vi "cluster2array_side_circle_overlay.vi"(10 "radius":i32, 11 "giltch of clusters":cluster{"giltch_coord":dbl[]}[](array[cluster])) -> (0 "Left side points":T1, 1 "Bottom side points":T1, 2 "Right side points":T1, 3 "Top side points":T1)   [LabVIEW 2017]
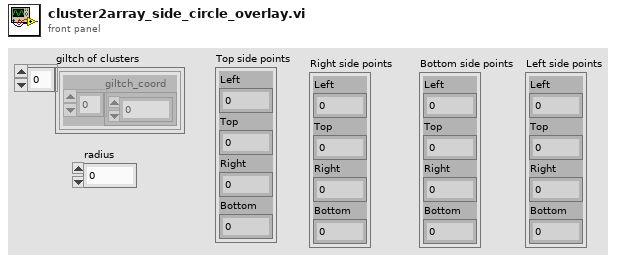
[diagram p1: front panel]
types:
  T1 = cluster{"Left":i32, "Top":i32, "Right":i32, "Bottom":i32}
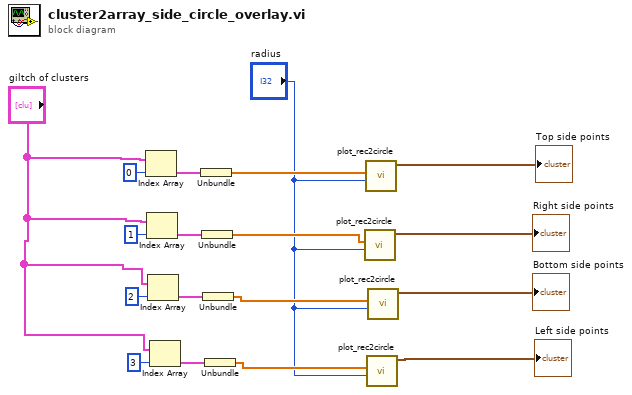
[diagram p0: block diagram]
diagram:
  n1 = Index Array(array="giltch of clusters", index=0 ("index (page)")) -> (element=w17:cluster{"giltch_coord":dbl[]})
  n2 = Index Array(array="giltch of clusters", index=1 ("index (page)")) -> (element=w14:cluster{"giltch_coord":dbl[]})
  n3 = Index Array(array="giltch of clusters", index=2 ("index (page)")) -> (element=w13:cluster{"giltch_coord":dbl[]})
  n4 = Index Array(array="giltch of clusters", index=3 ("index (page)")) -> (element=w10:cluster{"giltch_coord":dbl[]})
  n5 = Unbundle(w17) -> ("giltch_coord"=w8:dbl[])
  n6 = Unbundle(w14) -> ("giltch_coord"=w7:dbl[])
  n7 = Unbundle(w13) -> ("giltch_coord"=w6:dbl[])
  n8 = Unbundle(w10) -> ("giltch_coord"=w5:dbl[])
  n9 = call "plot_rec2circle.vi"("radius"="radius", "center of circle"=w7) -> ("data out"=→"Right side points":T1)  [unwired: 9 in]
  n10 = call "plot_rec2circle.vi"("radius"="radius", "center of circle"=w8) -> ("data out"=→"Top side points":T1)  [unwired: 9 in]
  n11 = call "plot_rec2circle.vi"("radius"="radius", "center of circle"=w5) -> ("data out"=→"Left side points":T1)  [unwired: 9 in]
  n12 = call "plot_rec2circle.vi"("radius"="radius", "center of circle"=w6) -> ("data out"=→"Bottom side points":T1)  [unwired: 9 in]
